vi "Cov_CO2.vi"(11 "Input x":dbl) -> (3 "CO2":dbl)   [LabVIEW 2011]
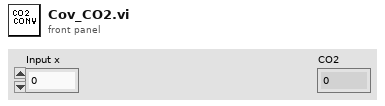
[diagram p1: front panel]
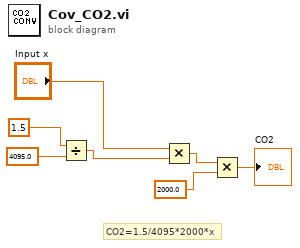
[diagram p0: block diagram]
diagram:
  # "CO2=1.5/4095*2000*x"
  n1 = Divide(x=1.5, y=4095.0) -> (x/y=w3:dbl)
  n2 = Multiply(x="Input x", y=w3) -> (x*y=w5:dbl)
  n3 = Multiply(x=w5, y=2000.0) -> (x*y=→"CO2":dbl)
